vi "Open System Definition File.vi"(8 "error in":errorcluster, 11 "path":path) -> (0 "error out":errorcluster, 1 "target ref":refnum<k24>, 2 "root ref":refnum<k24>, 3 "system definition ref":refnum<k24>)   [LabVIEW 2026]
uses:
  NationalInstruments.VeriStand.SystemDefinitionAPI
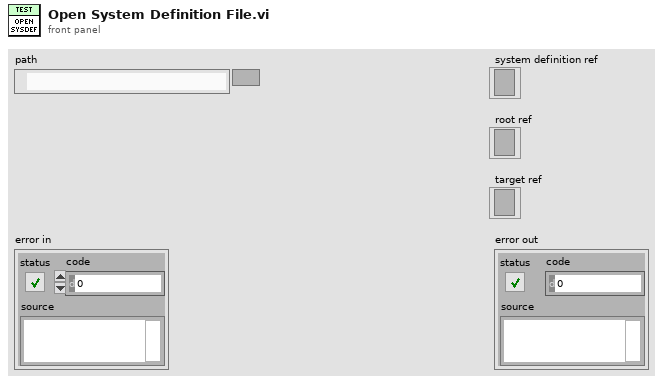
[diagram p1: front panel]
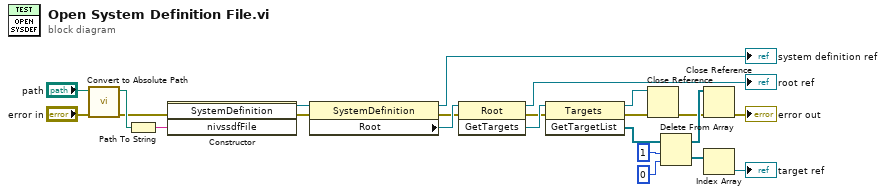
[diagram p0: block diagram]
diagram:
  n1 = call "Convert to Absolute Path.vi"("error in"="error in", "path"="path") -> ("error out"=w6:errorcluster, "absolute path"=w8:path)  [unwired: 8 in]
  n2 = Path To String(path=w8) -> (string=w7:string)
  n3 = constructor class="SystemDefinition"(error in=w6, "nivssdfFile"=w7) -> (reference out=w3:refnum<k24>, error out=w5:errorcluster)  [unwired: 2 in, 2 out]
  n4 = property class="SystemDefinition"(reference=w3, error in=w5) -> (reference out=→"system definition ref":refnum<k24>, error out=w21:errorcluster, "Root"=w23:refnum<k24>)
  n5 = invoke class="Root" method="GetTargets"(reference=w23, error in=w21) -> (reference out=→"root ref":refnum<k24>, error out=w20:errorcluster, "GetTargets"=w22:refnum<k24>)  [unwired: 1 in]
  n6 = invoke class="Targets" method="GetTargetList"(reference=w22, error in=w20) -> (reference out=w14:refnum<k24>, error out=w15:errorcluster, "GetTargetList"=w18:refnum<k24>[])  [unwired: 1 in]
  n7 = Close Reference(reference=w14, error in (no error)=w15) -> (error out=w11:errorcluster)
  n8 = Delete From Array(array=w18, length=1, index=0) -> (deleted portion=w2:refnum<k24>[], array with subset deleted=w12:refnum<k24>[])
  n9 = Close Reference(reference=w12, error in (no error)=w11) -> (error out=→"error out":errorcluster)
  n10 = Index Array(array=w2) -> (element=→"target ref":refnum<k24>)  [unwired: 1 in]
